vi "p01histograma.vi"() -> ()   [LabVIEW 2013]
panel:
  in  "Vertical Pointer Slide":dbl(slide) scale=0.0..10.0
  out "Waveform Graph":dbl[][](graph)
  out "2D Picture 2":picture
  out "2D Picture":picture
  in  "path to BMP file":path
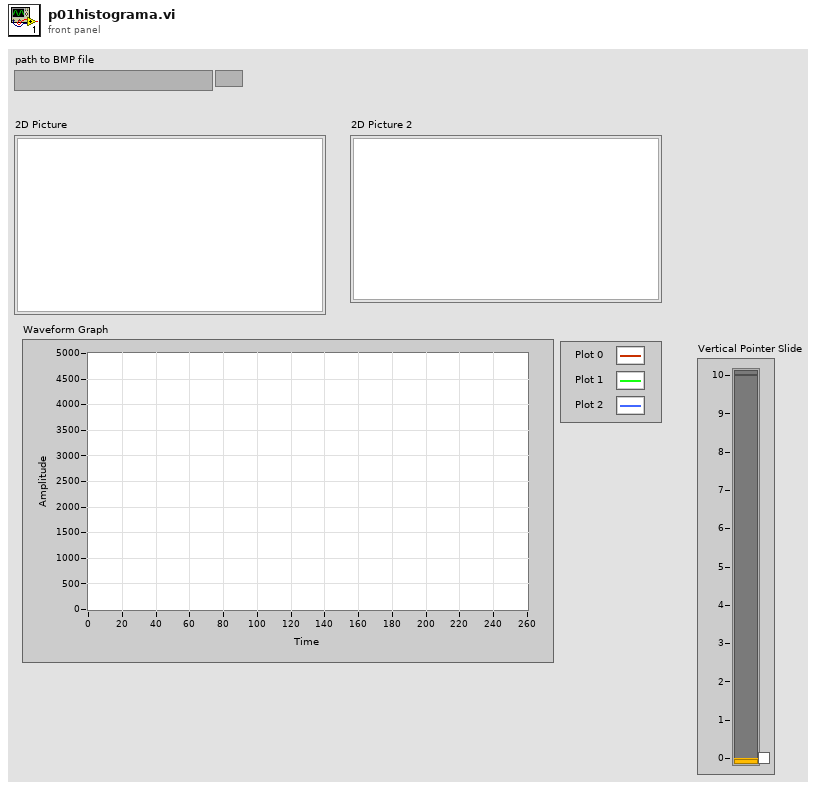
[diagram p1: front panel]
types:
  T1 = typedef "imagedata.ctl" = cluster{"image type":i32, "image depth":i32, "image":u8[], "mask":u8[], "colors":u32[], "Rectangle":cluster{"left":i16, "top":i16, "right":i16, "bottom":i16}}
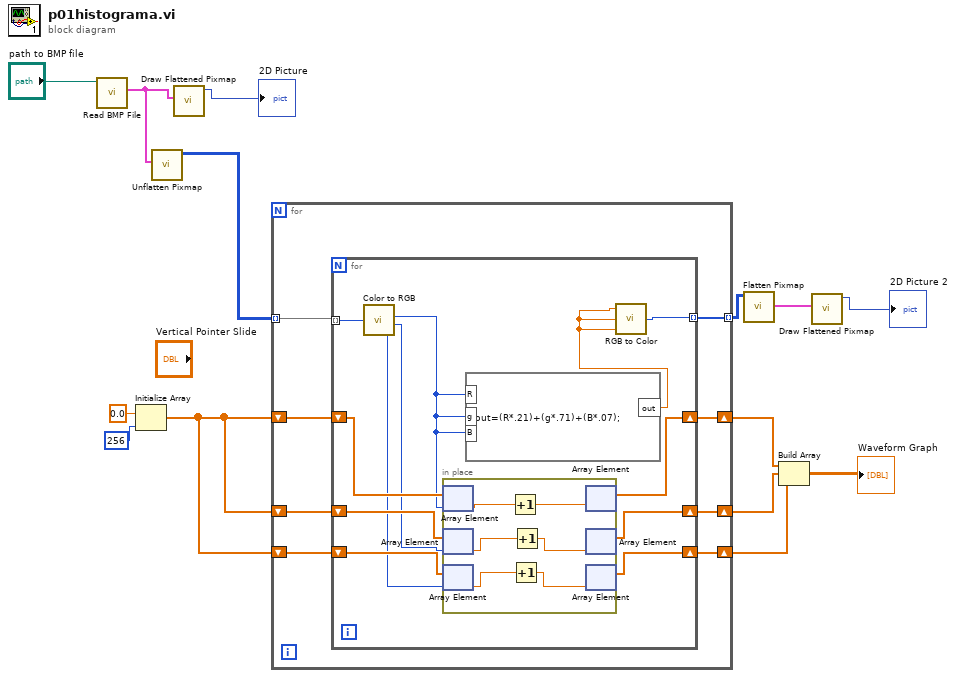
[diagram p0: block diagram]
diagram:
  n1 = call <vilib>:"Read BMP File.vi"("path to BMP file"="path to BMP file") -> ("image data"=w12:T1)  [unwired: 8 in, 2 out]
  n2 = Initialize Array(0.0 ("element"), 256 ("dimension size")) -> (w5:dbl[])
  n3 = call <vilib>:"Unflatten Pixmap.vi"("image data"=w12) -> ("24-bit pixmap"=w11:u32[][])  [unwired: 4 in, 6 out]
  n4 = call <vilib>:"Draw Flattened Pixmap.vi"("image data"=w12) -> ("new picture"=→"2D Picture":picture)  [unwired: 8 in]
  n5 = for {
    tunnel: w11 -> [w22] mode=indexing
    tunnel: [w21] -> w10 mode=indexing
    shift-right: [w19] -> w4
    shift-left: w5 -> [w20]
    shift-right: [w16] -> w3
    shift-left: w5 -> [w18]
    shift-right: [w15] -> w2
    shift-left: w5 -> [w17]
    n6 = for {
      tunnel: w22 -> [w34] mode=indexing
      tunnel: [w33] -> w21 mode=indexing
      shift-right: [w30] -> w19
      shift-left: w20 -> [w31]
      shift-right: [w27] -> w16
      shift-left: w18 -> [w29]
      shift-right: [w26] -> w15
      shift-left: w17 -> [w28]
      n7 = call <vilib>:"Color to RGB.vi"("Color"=w34) -> ("R"=w23:u8, "G"=w25:u8, "B"=w24:u8)  [unwired: 1 out]
      n8 = in-place {
        n9 = in-place-array #1(w31, w23) -> (w40:dbl)
        n10 = in-place-array #2(w29, w25) -> (w38:dbl)
        n11 = in-place-array #3(w28, w24) -> (w37:dbl)
        n12 = Increment(x=w40) -> (x+1=w39:dbl)
        n13 = Increment(x=w37) -> (x+1=w35:dbl)
        n14 = Increment(x=w38) -> (x+1=w36:dbl)
        n15 = in-place-array #1(w39) -> (w30:dbl[])  [unwired: 1 out]
        n16 = in-place-array #2(w36) -> (w27:dbl[])  [unwired: 1 out]
        n17 = in-place-array #3(w35) -> (w26:dbl[])  [unwired: 1 out]
      }
      n18 = formula code="out=(R*.21)+(g*.71)+(B*.07);"("R"=w23, "B"=w23, "g"=w23) -> ("out"=w32:dbl)
      n19 = call <vilib>:"RGB to Color.vi"("B"=w32, "G"=w32, "R"=w32) -> ("Color"=w33:u32)
    }
  }
  n20 = call <vilib>:"Flatten Pixmap.vi"("24-bit pixmap"=w10) -> ("image data"=w9:T1)  [unwired: 10 in]
  n21 = Build Array(w4, w3, w2) -> (→"Waveform Graph":dbl[][])
  n22 = call <vilib>:"Draw Flattened Pixmap.vi"("image data"=w9) -> ("new picture"=→"2D Picture 2":picture)  [unwired: 8 in]
